vi "Result_Test.vi"(8 "error in (no error)":errorcluster caption="entrée d'erreur (pas d'erreur)", 11 "Delay en entrée":refnum<class "additional_information_generation_SIN.lvclass">) -> (0 "error out":errorcluster caption="sortie d'erreur", 3 "Delay en sortie":refnum<class "additional_information_generation_SIN.lvclass">)   [LabVIEW 2020, in "Library Test.lvlib" / "additional_information_generation_SIN.lvclass"]
uses:
  additional_information_generation_SIN.lvclass
  Test_Without_Instr/Test_Without_Inst.lvclass
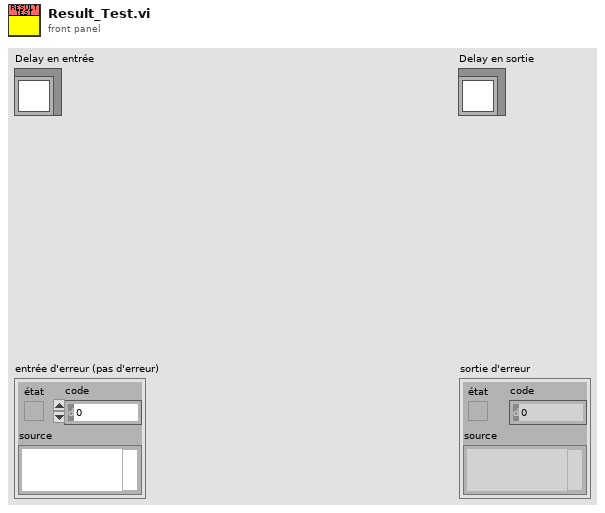
[diagram p1: front panel]
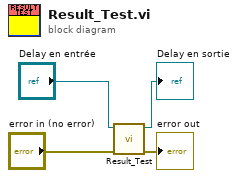
[diagram p0: block diagram]
diagram:
  n1 = call-parent "Result_Test.vi"("error in (no error)"="error in (no error)", "Test_Without_Inst en entrée"="Delay en entrée") -> ("error out"=→"error out":errorcluster, "Test_Without_Inst en sortie"=→"Delay en sortie":refnum<class "additional_information_generation_SIN.lvclass">)  [unwired: 8 in]
